vi "HEWH Standard Test Locations.vi"(7 "Test Data Path":path=path "C:/Users/220038920/Desktop/TestSeqSave.csv", 8 "error in (no error)":errorcluster, 11 "Test Name":string) -> (0 "error out":errorcluster, 3 "appended path":path)   [LabVIEW 2020]
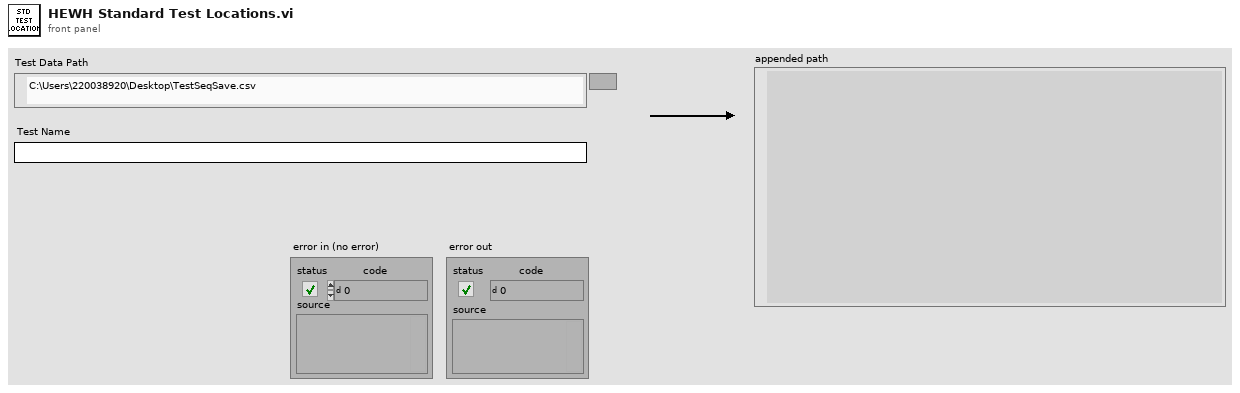
[diagram p1: front panel]
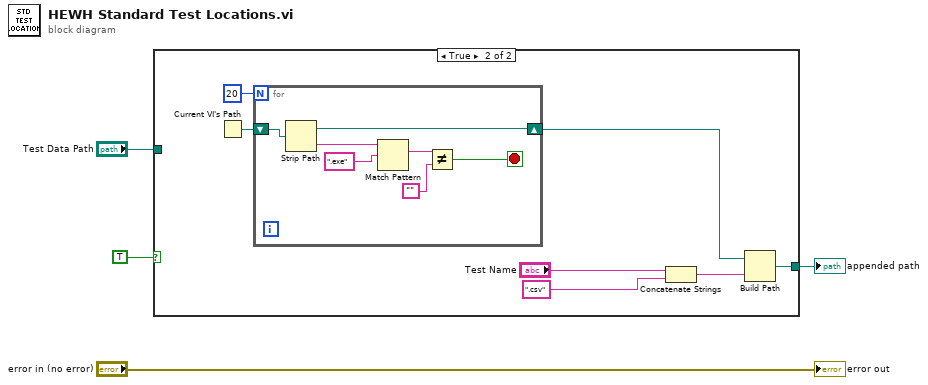
[diagram p0: block diagram]
diagram:
  n1 = case shown="True" TRUE {
    tunnel: [w5 w12] -> w4
    tunnel: "Test Data Path" -> [w5 _]
    frame False {
    }
    frame True {
      n2 = Current VI's Path() -> (path=w6:path)
      n3 = for {
        N: 20 -> [_]
        shift-right: [w18] -> w8
        shift-left: w6 -> [w19]
        stop <- w15 stop-if-true
        n4 = Strip Path(path=w19) -> (stripped path=w18:path, name=w14:string)
        n5 = Match Pattern(string=w14, regular expression=".exe" ("string")) -> (match substring=w17:string)  [unwired: 1 in, 3 out]
        n6 = Not Equal?(x=w17, y="") -> (x != y?=w15:bool)
      }
      n7 = Concatenate Strings("Test Name", ".csv" ("string")) -> (w9:string)
      n8 = Build Path(base path=w8, name or relative path=w9) -> (appended path=w12:path)
    }
  }
  "appended path" <- w4
  "error out" <- "error in (no error)"
